vi "HandleStopSync.vi"(8 "error in (no error)":errorcluster, 11 "S4GUI in":refnum<class "S4GUI.lvclass">) -> (0 "error out":errorcluster, 3 "S4GUI out":refnum<class "S4GUI.lvclass">)   [LabVIEW 2018, in "S4GUI.lvclass"]
uses:
  S4GUI.lvclass
  S4GUI.lvclass/S4GUI.ctl
  Instrument/Instrument.lvclass/Instrument.ctl
  Acquisition/Acquisition.lvclass
  Instrument/Instrument.lvclass
  Device/Optics/Opt_Selector/Opt_Selector.lvclass
  Channel/Channel.lvclass
  Interface/Interface.lvclass
  StateMachine/State Machine.lvclass
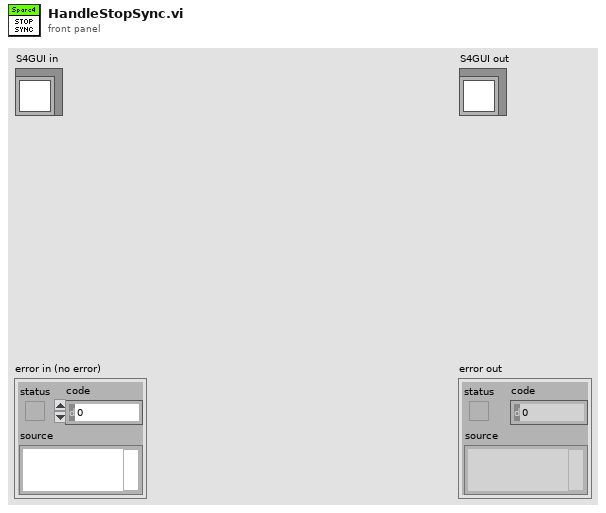
[diagram p1: front panel]
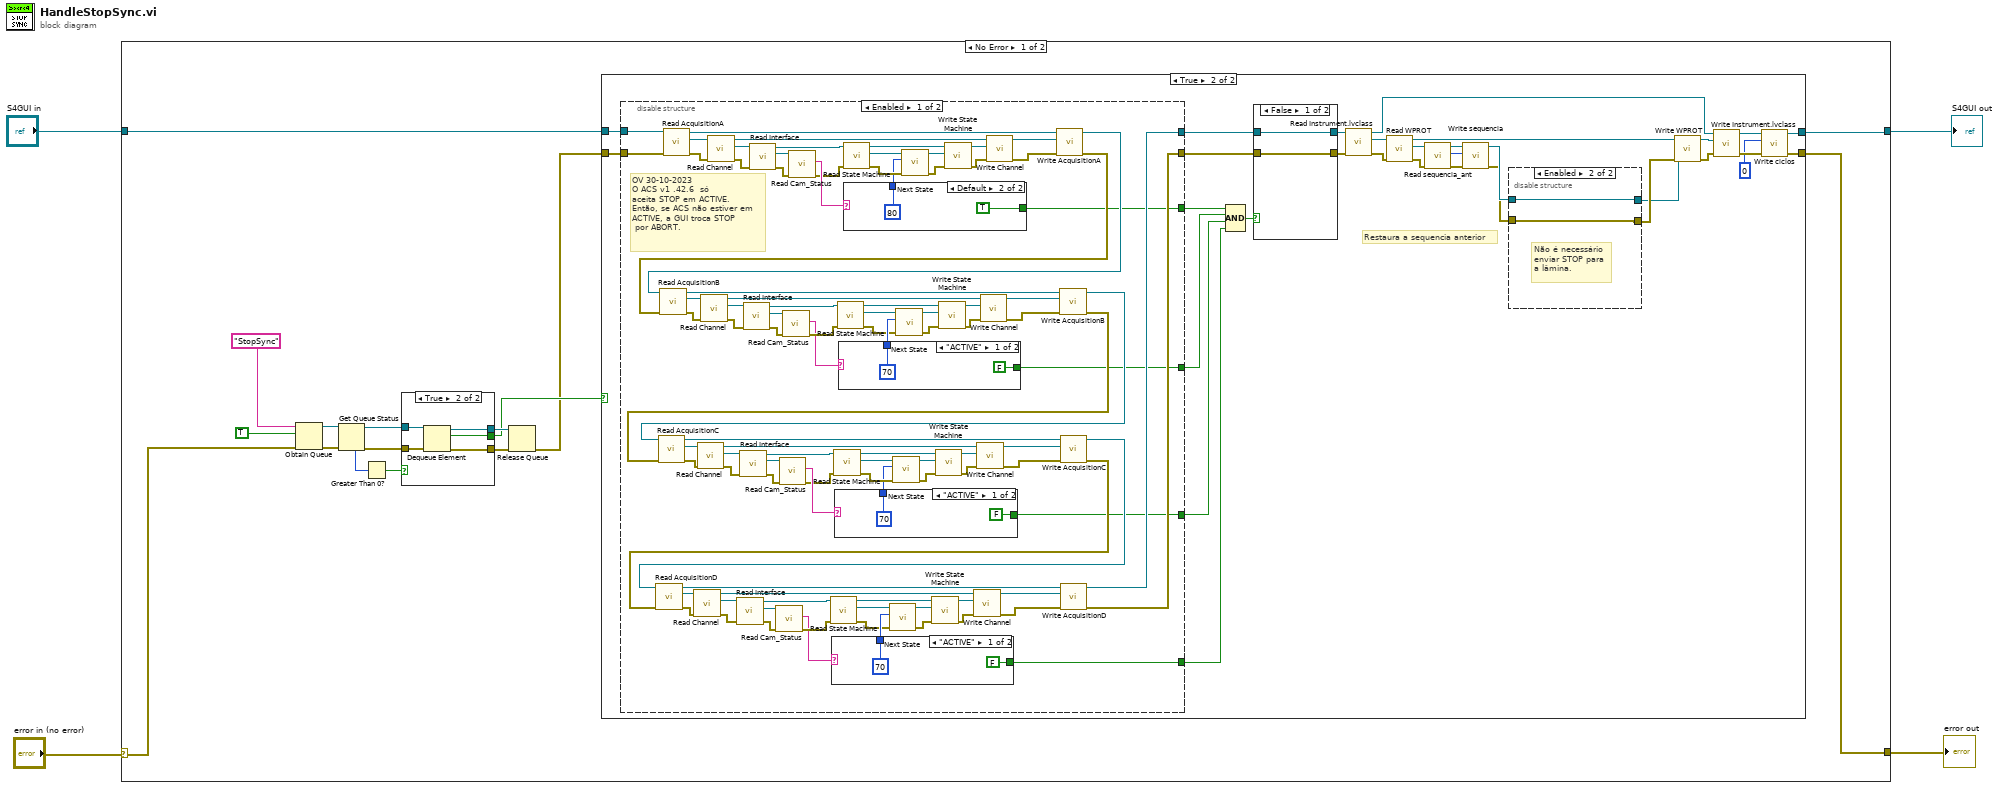
[diagram p0: block diagram]
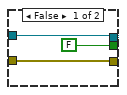
[diagram p2: hidden frame]
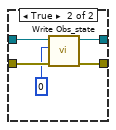
[diagram p4: hidden frame]
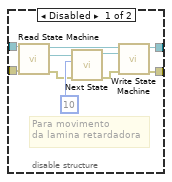
[diagram p5: hidden frame]
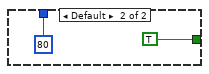
[diagram p6: hidden frame]
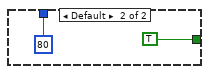
[diagram p7: hidden frame]
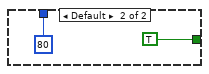
[diagram p8: hidden frame]
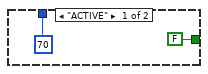
[diagram p9: hidden frame]
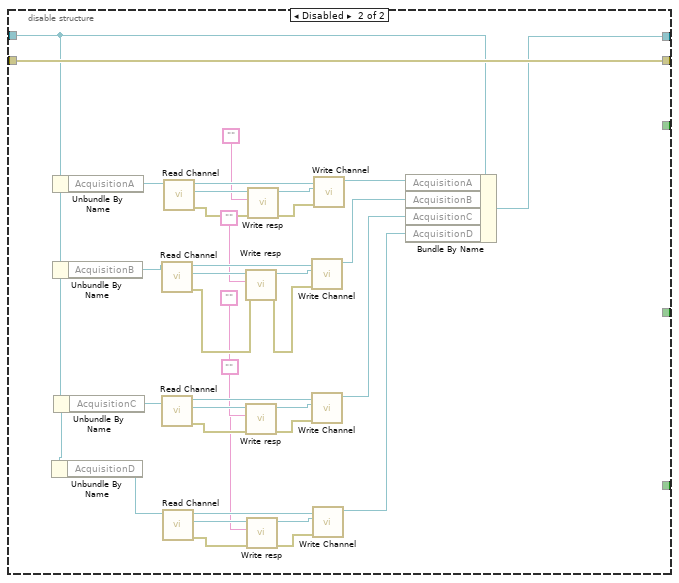
[diagram p10: hidden frame]
diagram:
  n1 = case shown="No Error" "error in (no error)" {
    selector: "error in (no error)" -> [w7 w231]
    tunnel: [w6 w231] -> w3
    tunnel: [w5 w230] -> w1
    tunnel: "S4GUI in" -> [w8 w230]
    frame No Error {
      n2 = Obtain Queue(name (unnamed)="StopSync", element data type=TRUE, error in (no error)=w7) -> (queue out=w17:refnum<queue>, error out=w18:errorcluster)  [unwired: 2 in, 1 out]
      n3 = Get Queue Status(queue=w17, error in (no error)=w18) -> (queue out=w14:refnum<queue>, error out=w13:errorcluster, # elements in queue=w16:i32)  [unwired: 1 in, 5 out]
      n4 = Greater Than 0?(x=w16) -> (x > 0?=w15:bool)
      n5 = case shown="True" w15 {
        tunnel: w14 -> [w22 w27]
        tunnel: w13 -> [w21 w28]
        tunnel: [FALSE w26] -> w10
        tunnel: [w22 w25] -> w12
        tunnel: [w21 w24] -> w11
        frame False {
        }
        frame True {
          n6 = Dequeue Element(queue=w27, error in (no error)=w28) -> (queue out=w25:refnum<queue>, element=w26:bool, error out=w24:errorcluster)  [unwired: 1 in, 1 out]
        }
      }
      n7 = Release Queue(queue=w12, error in (no error)=w11) -> (error out=w9:errorcluster)  [unwired: 1 in, 2 out]
      n8 = case shown="True" w10 {
        tunnel: w9 -> [w29 w59]
        tunnel: w8 -> [w30 w58]
        tunnel: [w29 w36] -> w6
        tunnel: [w30 w37] -> w5
        frame False {
        }
        frame True {
          # "Restaura a sequencia anterior"
          n9 = disable-structure shown="Enabled" {
            disable-tunnel: [w154 w228] -> w61
            disable-tunnel: [w153 w229] -> w60
            disable-tunnel: w59 -> [w152 w229]
            disable-tunnel: w58 -> [w151 w201]
            disable-tunnel: [w143 _] -> w34
            disable-tunnel: [w123 _] -> w33
            disable-tunnel: [w103 _] -> w32
            disable-tunnel: [w82 _] -> w31
            frame Enabled {
              # "OV 30-10-2023\nO ACS v1 .42.6  só\naceita STOP em ACTIVE.\nEntão, se ACS não estiver em \nACTIVE, a GUI troca STOP\n por ABORT."
              n10 = call-dynamic "Read AcquisitionA.vi"("error in (no error)"=w152, "S4ACS_GUI in"=w151) -> ("error out"=w168:errorcluster, "Acquisition.lvclass"=w167:refnum<class "Acquisition.lvclass">, "S4ACS_GUI out"=w165:refnum<class "S4GUI.lvclass">)  [unwired: 7 in]
              n11 = call-dynamic "Read Channel.vi"("error in (no error)"=w168, "Acquisition in"=w167) -> ("error out"=w149:errorcluster, "Channel.lvclass"=w150:refnum<class "Channel.lvclass">, "Acquisition out"=w176:refnum<class "Acquisition.lvclass">)  [unwired: 7 in]
              n12 = call-dynamic "Read Interface.vi"("error in (no error)"=w149, "Channel in"=w150) -> ("error out"=w146:errorcluster, "Interface.lvclass"=w147:refnum<class "Interface.lvclass">, "Channel out"=w148:refnum<class "Channel.lvclass">)  [unwired: 7 in]
              n13 = call-dynamic "Read Cam_Status.vi"("error in (no error)"=w146, "Interface in"=w147) -> ("error out"=w144:errorcluster, "Cam_Status"=w145:string)  [unwired: 7 in, 1 out]
              n14 = call-dynamic "Read State Machine.vi"("error in (no error)"=w144, "Device in"=w148) -> ("error out"=w170:errorcluster, "State Machine.lvclass"=w169:refnum<class "State Machine.lvclass">, "Device out"=w172:refnum<class "Channel.lvclass">)  [unwired: 7 in]
              n15 = case shown="Default" w145 {
                tunnel: [70 80] -> w166
                tunnel: [FALSE TRUE] -> w143
                frame "ACTIVE" {
                }
                frame Default {
                }
              }
              n16 = call "Next State.vi"("error in (no error)"=w170, "New_State"=w166, "State Machine in"=w169) -> ("error out"=w173:errorcluster, "State Machine out"=w171:refnum<class "State Machine.lvclass">)  [unwired: 7 in]
              n17 = call-dynamic "Write State Machine.vi"("error in (no error)"=w173, "State Machine.lvclass"=w171, "Device in"=w172) -> ("error out"=w177:errorcluster, "Device out"=w178:refnum<class "Channel.lvclass">)  [unwired: 7 in]
              n18 = call-dynamic "Write Channel.vi"("error in (no error)"=w177, "Channel.lvclass"=w178, "Acquisition in"=w176) -> ("error out"=w175:errorcluster, "Acquisition out"=w174:refnum<class "Acquisition.lvclass">)  [unwired: 7 in]
              n19 = call-dynamic "Write AcquisitionA.vi"("error in (no error)"=w175, "Acquisition.lvclass"=w174, "S4ACS_GUI in"=w165) -> ("error out"=w164:errorcluster, "S4ACS_GUI out"=w163:refnum<class "S4GUI.lvclass">)  [unwired: 7 in]
              n20 = call "Read AcquisitionB.vi"("error in (no error)"=w164, "S4ACS_GUI in"=w163) -> ("error out"=w161:errorcluster, "Acquisition.lvclass"=w162:refnum<class "Acquisition.lvclass">, "S4ACS_GUI out"=w129:refnum<class "S4GUI.lvclass">)  [unwired: 7 in]
              n21 = call-dynamic "Read Channel.vi"("error in (no error)"=w161, "Acquisition in"=w162) -> ("error out"=w125:errorcluster, "Channel.lvclass"=w124:refnum<class "Channel.lvclass">, "Acquisition out"=w127:refnum<class "Acquisition.lvclass">)  [unwired: 7 in]
              n22 = call-dynamic "Read Interface.vi"("error in (no error)"=w125, "Channel in"=w124) -> ("error out"=w140:errorcluster, "Interface.lvclass"=w139:refnum<class "Interface.lvclass">, "Channel out"=w138:refnum<class "Channel.lvclass">)  [unwired: 7 in]
              n23 = call-dynamic "Read Cam_Status.vi"("error in (no error)"=w140, "Interface in"=w139) -> ("error out"=w142:errorcluster, "Cam_Status"=w141:string)  [unwired: 7 in, 1 out]
              n24 = call-dynamic "Read State Machine.vi"("error in (no error)"=w142, "Device in"=w138) -> ("error out"=w135:errorcluster, "State Machine.lvclass"=w136:refnum<class "State Machine.lvclass">, "Device out"=w133:refnum<class "Channel.lvclass">)  [unwired: 7 in]
              n25 = case shown="\"ACTIVE\"" w141 {
                tunnel: [70 80] -> w137
                tunnel: [FALSE TRUE] -> w123
                frame "ACTIVE" {
                }
                frame Default {
                }
              }
              n26 = call "Next State.vi"("error in (no error)"=w135, "New_State"=w137, "State Machine in"=w136) -> ("error out"=w132:errorcluster, "State Machine out"=w134:refnum<class "State Machine.lvclass">)  [unwired: 7 in]
              n27 = call-dynamic "Write State Machine.vi"("error in (no error)"=w132, "State Machine.lvclass"=w134, "Device in"=w133) -> ("error out"=w131:errorcluster, "Device out"=w130:refnum<class "Channel.lvclass">)  [unwired: 7 in]
              n28 = call-dynamic "Write Channel.vi"("error in (no error)"=w131, "Channel.lvclass"=w130, "Acquisition in"=w127) -> ("error out"=w126:errorcluster, "Acquisition out"=w128:refnum<class "Acquisition.lvclass">)  [unwired: 7 in]
              n29 = call "Write AcquisitionB.vi"("error in (no error)"=w126, "Acquisition.lvclass"=w128, "S4ACS_GUI in"=w129) -> ("error out"=w158:errorcluster, "S4ACS_GUI out"=w157:refnum<class "S4GUI.lvclass">)  [unwired: 7 in]
              n30 = call-dynamic "Read AcquisitionC.vi"("error in (no error)"=w158, "S4ACS_GUI in"=w157) -> ("error out"=w104:errorcluster, "Acquisition.lvclass"=w81:refnum<class "Acquisition.lvclass">, "S4ACS_GUI out"=w160:refnum<class "S4GUI.lvclass">)  [unwired: 7 in]
              n31 = call-dynamic "Read Channel.vi"("error in (no error)"=w104, "Acquisition in"=w81) -> ("error out"=w121:errorcluster, "Channel.lvclass"=w122:refnum<class "Channel.lvclass">, "Acquisition out"=w120:refnum<class "Acquisition.lvclass">)  [unwired: 7 in]
              n32 = call-dynamic "Read Interface.vi"("error in (no error)"=w121, "Channel in"=w122) -> ("error out"=w109:errorcluster, "Interface.lvclass"=w110:refnum<class "Interface.lvclass">, "Channel out"=w111:refnum<class "Channel.lvclass">)  [unwired: 7 in]
              n33 = call-dynamic "Read Cam_Status.vi"("error in (no error)"=w109, "Interface in"=w110) -> ("error out"=w107:errorcluster, "Cam_Status"=w108:string)  [unwired: 7 in, 1 out]
              n34 = call-dynamic "Read State Machine.vi"("error in (no error)"=w107, "Device in"=w111) -> ("error out"=w114:errorcluster, "State Machine.lvclass"=w113:refnum<class "State Machine.lvclass">, "Device out"=w116:refnum<class "Channel.lvclass">)  [unwired: 7 in]
              n35 = case shown="\"ACTIVE\"" w108 {
                tunnel: [70 80] -> w112
                tunnel: [FALSE TRUE] -> w103
                frame "ACTIVE" {
                }
                frame Default {
                }
              }
              n36 = call "Next State.vi"("error in (no error)"=w114, "New_State"=w112, "State Machine in"=w113) -> ("error out"=w117:errorcluster, "State Machine out"=w115:refnum<class "State Machine.lvclass">)  [unwired: 7 in]
              n37 = call-dynamic "Write State Machine.vi"("error in (no error)"=w117, "State Machine.lvclass"=w115, "Device in"=w116) -> ("error out"=w118:errorcluster, "Device out"=w119:refnum<class "Channel.lvclass">)  [unwired: 7 in]
              n38 = call-dynamic "Write Channel.vi"("error in (no error)"=w118, "Channel.lvclass"=w119, "Acquisition in"=w120) -> ("error out"=w105:errorcluster, "Acquisition out"=w106:refnum<class "Acquisition.lvclass">)  [unwired: 7 in]
              n39 = call-dynamic "Write AcquisitionC.vi"("error in (no error)"=w105, "Acquisition.lvclass"=w106, "S4ACS_GUI in"=w160) -> ("error out"=w156:errorcluster, "S4ACS_GUI out"=w155:refnum<class "S4GUI.lvclass">)  [unwired: 7 in]
              n40 = call-dynamic "Read AcquisitionD.vi"("error in (no error)"=w156, "S4ACS_GUI in"=w155) -> ("error out"=w83:errorcluster, "Acquisition.lvclass"=w84:refnum<class "Acquisition.lvclass">, "S4ACS_GUI out"=w159:refnum<class "S4GUI.lvclass">)  [unwired: 7 in]
              n41 = call-dynamic "Read Channel.vi"("error in (no error)"=w83, "Acquisition in"=w84) -> ("error out"=w88:errorcluster, "Channel.lvclass"=w87:refnum<class "Channel.lvclass">, "Acquisition out"=w89:refnum<class "Acquisition.lvclass">)  [unwired: 7 in]
              n42 = call-dynamic "Read Interface.vi"("error in (no error)"=w88, "Channel in"=w87) -> ("error out"=w100:errorcluster, "Interface.lvclass"=w99:refnum<class "Interface.lvclass">, "Channel out"=w98:refnum<class "Channel.lvclass">)  [unwired: 7 in]
              n43 = call-dynamic "Read Cam_Status.vi"("error in (no error)"=w100, "Interface in"=w99) -> ("error out"=w102:errorcluster, "Cam_Status"=w101:string)  [unwired: 7 in, 1 out]
              n44 = call-dynamic "Read State Machine.vi"("error in (no error)"=w102, "Device in"=w98) -> ("error out"=w95:errorcluster, "State Machine.lvclass"=w96:refnum<class "State Machine.lvclass">, "Device out"=w93:refnum<class "Channel.lvclass">)  [unwired: 7 in]
              n45 = case shown="\"ACTIVE\"" w101 {
                tunnel: [70 80] -> w97
                tunnel: [FALSE TRUE] -> w82
                frame "ACTIVE" {
                }
                frame Default {
                }
              }
              n46 = call "Next State.vi"("error in (no error)"=w95, "New_State"=w97, "State Machine in"=w96) -> ("error out"=w92:errorcluster, "State Machine out"=w94:refnum<class "State Machine.lvclass">)  [unwired: 7 in]
              n47 = call-dynamic "Write State Machine.vi"("error in (no error)"=w92, "State Machine.lvclass"=w94, "Device in"=w93) -> ("error out"=w91:errorcluster, "Device out"=w90:refnum<class "Channel.lvclass">)  [unwired: 7 in]
              n48 = call-dynamic "Write Channel.vi"("error in (no error)"=w91, "Channel.lvclass"=w90, "Acquisition in"=w89) -> ("error out"=w85:errorcluster, "Acquisition out"=w86:refnum<class "Acquisition.lvclass">)  [unwired: 7 in]
              n49 = call-dynamic "Write AcquisitionD.vi"("error in (no error)"=w85, "Acquisition.lvclass"=w86, "S4ACS_GUI in"=w159) -> ("error out"=w153:errorcluster, "S4ACS_GUI out"=w154:refnum<class "S4GUI.lvclass">)  [unwired: 7 in]
            }
            frame Disabled {
              n50 = Unbundle By Name(w201) -> ("AcquisitionD"=w198:refnum<class "Acquisition.lvclass">)
              n51 = Unbundle By Name(w201) -> ("AcquisitionA"=w227:refnum<class "Acquisition.lvclass">)
              n52 = Unbundle By Name(w201) -> ("AcquisitionB"=w200:refnum<class "Acquisition.lvclass">)
              n53 = Unbundle By Name(w201) -> ("AcquisitionC"=w199:refnum<class "Acquisition.lvclass">)
              n54 = call-dynamic "Read Channel.vi"("Acquisition in"=w200) -> ("error out"=w216:errorcluster, "Channel.lvclass"=w218:refnum<class "Channel.lvclass">, "Acquisition out"=w219:refnum<class "Acquisition.lvclass">)  [unwired: 8 in]
              n55 = call-dynamic "Read Channel.vi"("Acquisition in"=w199) -> ("error out"=w210:errorcluster, "Channel.lvclass"=w212:refnum<class "Channel.lvclass">, "Acquisition out"=w213:refnum<class "Acquisition.lvclass">)  [unwired: 8 in]
              n56 = call-dynamic "Read Channel.vi"("Acquisition in"=w198) -> ("error out"=w204:errorcluster, "Channel.lvclass"=w206:refnum<class "Channel.lvclass">, "Acquisition out"=w207:refnum<class "Acquisition.lvclass">)  [unwired: 8 in]
              n57 = call-dynamic "Read Channel.vi"("Acquisition in"=w227) -> ("error out"=w222:errorcluster, "Channel.lvclass"=w225:refnum<class "Channel.lvclass">, "Acquisition out"=w226:refnum<class "Acquisition.lvclass">)  [unwired: 8 in]
              n58 = call-dynamic "Write resp.vi"("error in (no error)"=w216, "resp"="", "Device in"=w218) -> ("error out"=w215:errorcluster, "Device out"=w217:refnum<class "Channel.lvclass">)  [unwired: 7 in]
              n59 = call-dynamic "Write resp.vi"("error in (no error)"=w210, "resp"="", "Device in"=w212) -> ("error out"=w209:errorcluster, "Device out"=w211:refnum<class "Channel.lvclass">)  [unwired: 7 in]
              n60 = call-dynamic "Write resp.vi"("error in (no error)"=w204, "resp"="", "Device in"=w206) -> ("error out"=w203:errorcluster, "Device out"=w205:refnum<class "Channel.lvclass">)  [unwired: 7 in]
              n61 = call-dynamic "Write resp.vi"("error in (no error)"=w222, "resp"="", "Device in"=w225) -> ("error out"=w221:errorcluster, "Device out"=w224:refnum<class "Channel.lvclass">)  [unwired: 7 in]
              n62 = call-dynamic "Write Channel.vi"("error in (no error)"=w215, "Channel.lvclass"=w217, "Acquisition in"=w219) -> ("Acquisition out"=w197:refnum<class "Acquisition.lvclass">)  [unwired: 7 in, 1 out]
              n63 = call-dynamic "Write Channel.vi"("error in (no error)"=w209, "Channel.lvclass"=w211, "Acquisition in"=w213) -> ("Acquisition out"=w196:refnum<class "Acquisition.lvclass">)  [unwired: 7 in, 1 out]
              n64 = call-dynamic "Write Channel.vi"("error in (no error)"=w203, "Channel.lvclass"=w205, "Acquisition in"=w207) -> ("Acquisition out"=w195:refnum<class "Acquisition.lvclass">)  [unwired: 7 in, 1 out]
              n65 = call-dynamic "Write Channel.vi"("error in (no error)"=w221, "Channel.lvclass"=w224, "Acquisition in"=w226) -> ("Acquisition out"=w223:refnum<class "Acquisition.lvclass">)  [unwired: 7 in, 1 out]
              n66 = Bundle By Name(cluster=w201, "AcquisitionA"=w223, "AcquisitionB"=w197, "AcquisitionC"=w196, "AcquisitionD"=w195) -> (w228:refnum<class "S4GUI.lvclass">)
            }
          }
          n67 = Compound Arithmetic op=AND(w34, w33, w32, w31) -> (w35:bool)
          n68 = case shown="False" w35 {
            tunnel: w61 -> [w63 w68]
            tunnel: w60 -> [w62 w67]
            tunnel: [w63 w66] -> w39
            tunnel: [w62 w65] -> w38
            frame False {
            }
            frame True {
              n69 = call-dynamic "Write Obs_state.vi"("error in (no error)"=w67, "Obs_state"=u32 0, "S4ACS_GUI in"=w68) -> ("error out"=w65:errorcluster, "S4ACS_GUI out"=w66:refnum<class "S4GUI.lvclass">)  [unwired: 7 in]
            }
          }
          n70 = call "Read Instrument.lvclass.vi"("error in (no error)"=w38, "S4ACS_GUI in"=w39) -> ("error out"=w52:errorcluster, "Instrument.lvclass"=w54:refnum<class "Instrument.lvclass">, "S4ACS_GUI out"=w53:refnum<class "S4GUI.lvclass">)  [unwired: 7 in]
          n71 = call "Read WPROT.vi"("error in (no error)"=w52, "Instrument in"=w54) -> ("error out"=w47:errorcluster, "Opt_Selector.lvclass"=w50:refnum<class "Opt_Selector.lvclass">, "Instrument out"=w55:refnum<class "Instrument.lvclass">)  [unwired: 7 in]
          n72 = call-dynamic "Read sequencia_ant.vi"("error in (no error)"=w47, "Opt_Selector in"=w50) -> ("error out"=w46:errorcluster, "sequencia_ant"=w48:u16, "Opt_Selector out"=w49:refnum<class "Opt_Selector.lvclass">)  [unwired: 7 in]
          n73 = call-dynamic "Write sequencia.vi"("error in (no error)"=w46, "sequencia"=w48, "Opt_Selector in"=w49) -> ("error out"=w44:errorcluster, "Opt_Selector out"=w45:refnum<class "Opt_Selector.lvclass">)  [unwired: 7 in]
          n74 = disable-structure shown="Enabled" {
            disable-tunnel: w45 -> [w75 w80]
            disable-tunnel: w44 -> [w74 w79]
            disable-tunnel: [w70 w79] -> w43
            disable-tunnel: [w69 w80] -> w42
            frame Disabled {
              # "Para movimento \nda lamina retardadora"
              n75 = call-dynamic "Read State Machine.vi"("error in (no error)"=w74, "Device in"=w75) -> ("error out"=w77:errorcluster, "State Machine.lvclass"=w72:refnum<class "State Machine.lvclass">, "Device out"=w73:refnum<class "Opt_Selector.lvclass">)  [unwired: 7 in]
              n76 = call "Next State.vi"("error in (no error)"=w77, "New_State"=10, "State Machine in"=w72) -> ("error out"=w76:errorcluster, "State Machine out"=w71:refnum<class "State Machine.lvclass">)  [unwired: 7 in]
              n77 = call-dynamic "Write State Machine.vi"("error in (no error)"=w76, "State Machine.lvclass"=w71, "Device in"=w73) -> ("error out"=w70:errorcluster, "Device out"=w69:refnum<class "Opt_Selector.lvclass">)  [unwired: 7 in]
            }
            frame Enabled {
              # "Não é necessário\nenviar STOP para\na lâmina."
            }
          }
          n78 = call "Write WPROT.vi"("error in (no error)"=w43, "Opt_Selector.lvclass"=w42, "Instrument in"=w55) -> ("error out"=w40:errorcluster, "Instrument out"=w41:refnum<class "Instrument.lvclass">)  [unwired: 7 in]
          n79 = call "Write Instrument.lvclass.vi"("error in (no error)"=w40, "Instrument.lvclass"=w41, "S4ACS_GUI in"=w53) -> ("error out"=w56:errorcluster, "S4ACS_GUI out"=w57:refnum<class "S4GUI.lvclass">)  [unwired: 7 in]
          n80 = call-dynamic "Write ciclos.vi"("error in (no error)"=w56, "ciclos"=u32 0, "S4ACS_GUI in"=w57) -> ("error out"=w36:errorcluster, "S4ACS_GUI out"=w37:refnum<class "S4GUI.lvclass">)  [unwired: 7 in]
        }
      }
    }
    frame Error {
    }
  }
  "error out" <- w3
  "S4GUI out" <- w1
